vi "hex2bin.vi"() -> ()   [LabVIEW 2020]
panel:
  out "Numeric 2":u8 format="%08b"
  in  "Numeric":u8 format="%x"
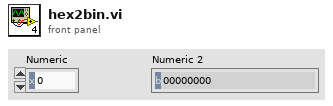
[diagram p1: front panel]
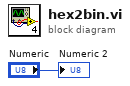
[diagram p0: block diagram]
diagram:
  "Numeric 2" <- "Numeric"
